vi "File.Find File in Folder using pattern.vi"(8 "error in (no error)":errorcluster, 10 "Pattern":string, 11 "Folder":path) -> (0 "error out":errorcluster, 3 "Found File":path)   [LabVIEW 2018]
uses:
  Errors/Error.Error Code List.ctl
  <vilib>/KATE/Files/File Utils.lvlib
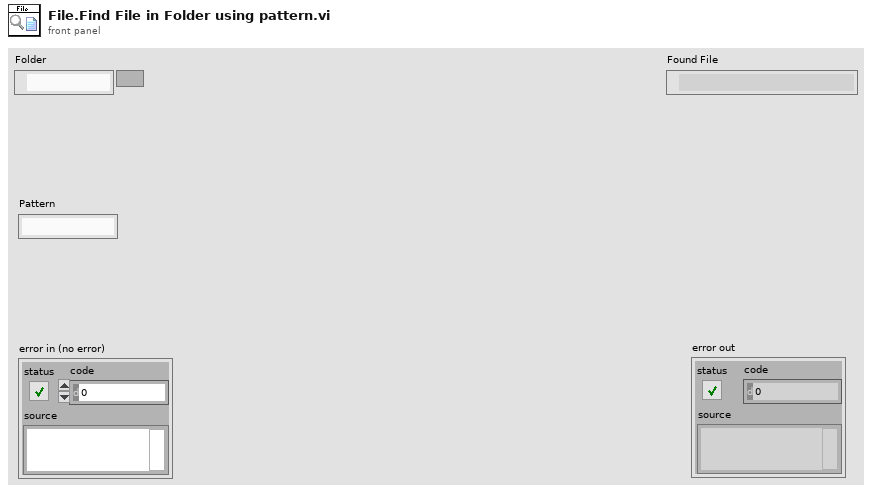
[diagram p1: front panel]
types:
  T1 = typedef "Error.Error Code List.ctl" = i32
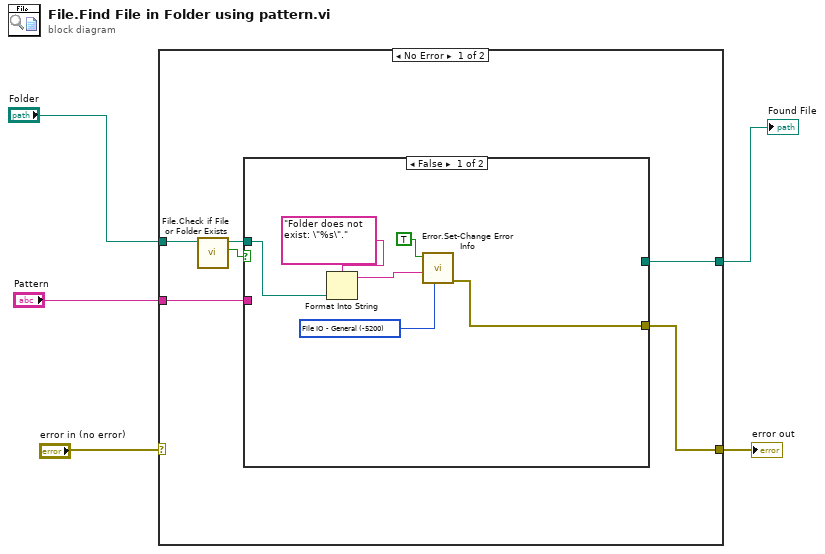
[diagram p0: block diagram]
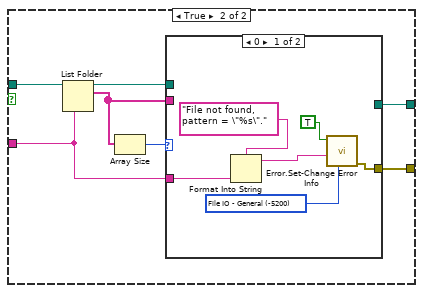
[diagram p2: hidden frame]
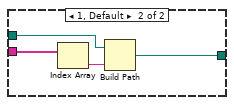
[diagram p3: hidden frame]
diagram:
  n1 = case shown="No Error" "error in (no error)" {
    selector: "error in (no error)" -> [_ w35]
    tunnel: "Folder" -> [w9 _]
    tunnel: [w11 _] -> w4
    tunnel: "Pattern" -> [w10 _]
    tunnel: [w6 w35] -> w1
    frame No Error {
      n2 = call <vilib>:"File.Check if File or Folder Exists.vi"("Path"=w9) -> ("Exists"=w7:bool, "Dup Path"=w8:path)  [unwired: 6 in, 3 out]
      n3 = case shown="False" w7 {
        tunnel: [_ w23] -> w11
        tunnel: w10 -> [_ w19]
        tunnel: w8 -> [w13 w22]
        tunnel: [w16 w18] -> w6
        frame False {
          w12 = T1 -5200 items=["No Error"=0, "Abort"=-2, "Misc"=-5000, "Fixture Error"=-5100, "File IO - General"=-5200, "FIle IO - Config Error"=-5201, "Instrument - General"=-5300, "Instrument - Serial Com"=-5301, "Instrument - Camera"=-5302, "Instrument - PS"=-5303, "Instrument - Oscilloscope"=-5304, "Instrument - Function Gen"=-5305, "Instrument - Load"=-5306, "Instrument - Meter"=-5307, "Instrument - Power Control"=-5308, "Instrument - Motion"=-5309, "Instrument - RF"=-5310, "System Exe"=-5400, "Image Processing"=-5500, "Communication"=-5600, "Script - Syntax Error"=-6000, "Script - Invalid Name or Param"=-6100, "Script - Timeout"=-6200, "Invalid Data"=-6300, "FW Update Error"=-6500] ("Std Code")
          n4 = Format Into String(format string="Folder does not exist: \"%s\"." ("Description"), w13) -> (resulting string=w14:string)  [unwired: 2 in, 1 out]
          n5 = call "Error.Set-Change Error Info.vi"("Std Code"=w12, "Description"=w14, "Set Error"=TRUE) -> ("error out"=w16:errorcluster)  [unwired: 8 in]
        }
        frame True {
          n6 = List Folder(path=w22, pattern=w19) -> (path out=w24:path, filenames=w21:string[])  [unwired: 2 in, 2 out]
          n7 = Array Size(array=w21) -> (size(s)=w20:i32)
          n8 = case shown="0" w20 {
            tunnel: w24 -> [_ w33]
            tunnel: [_ w32] -> w23
            tunnel: w21 -> [_ w31]
            tunnel: w19 -> [w27 _]
            tunnel: [w25 _] -> w18
            frame 0 {
              w26 = T1 -5200 items=["No Error"=0, "Abort"=-2, "Misc"=-5000, "Fixture Error"=-5100, "File IO - General"=-5200, "FIle IO - Config Error"=-5201, "Instrument - General"=-5300, "Instrument - Serial Com"=-5301, "Instrument - Camera"=-5302, "Instrument - PS"=-5303, "Instrument - Oscilloscope"=-5304, "Instrument - Function Gen"=-5305, "Instrument - Load"=-5306, "Instrument - Meter"=-5307, "Instrument - Power Control"=-5308, "Instrument - Motion"=-5309, "Instrument - RF"=-5310, "System Exe"=-5400, "Image Processing"=-5500, "Communication"=-5600, "Script - Syntax Error"=-6000, "Script - Invalid Name or Param"=-6100, "Script - Timeout"=-6200, "Invalid Data"=-6300, "FW Update Error"=-6500] ("Std Code")
              n9 = Format Into String(format string="File not found, pattern = \"%s\"." ("Description"), w27) -> (resulting string=w30:string)  [unwired: 2 in, 1 out]
              n10 = call "Error.Set-Change Error Info.vi"("Std Code"=w26, "Description"=w30, "Set Error"=TRUE) -> ("error out"=w25:errorcluster)  [unwired: 8 in]
            }
            frame 1, Default {
              n11 = Index Array(array=w31) -> (element=w34:string)  [unwired: 1 in]
              n12 = Build Path(base path=w33, name or relative path=w34) -> (appended path=w32:path)
            }
          }
        }
      }
    }
    frame Error {
    }
  }
  "Found File" <- w4
  "error out" <- w1
